vi "ParseMessage.vi"(11 "message in":string) -> (0 "Message type out":T1, 2 "Filename":string, 3 "message/data out":string)   [LabVIEW 2023, in "TCP_Server_Connection_Handler.lvlib" / "TCP_Server_Connection_Handler.lvclass"]
uses:
  TCP_Server_Connection_Handler.lvclass
  TCP_Server_Connection_Handler.lvclass/TCP_Server_Connection_Handler.ctl
  TypeDefinitions/messageType.ctl
  TCP_Server_Connection_Handler.lvlib
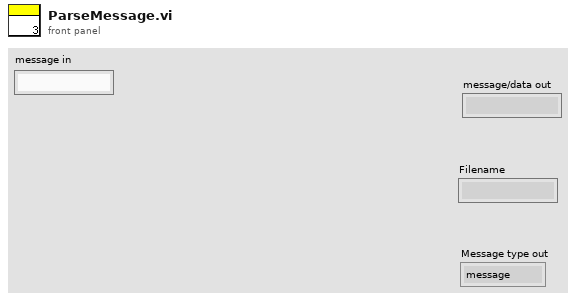
[diagram p1: front panel]
types:
  T1 = typedef "TCP_Server_Connection_Handler.lvlib/messageType.ctl" = enum16{"message", "file", "get", "ShutDown"}
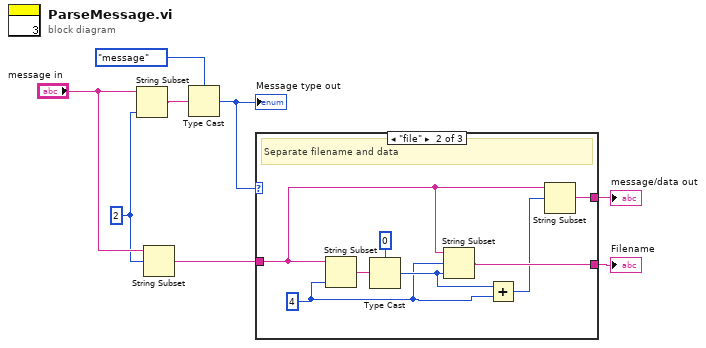
[diagram p0: block diagram]
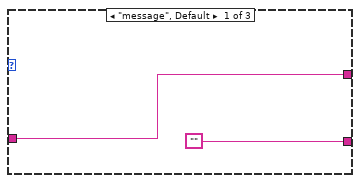
[diagram p2: hidden frame]
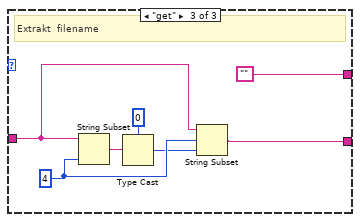
[diagram p3: hidden frame]
diagram:
  w2 = 2 ("length (rest)")
  n1 = String Subset(string="message in", length (rest)=w2) -> (substring=w5:string)  [unwired: 1 in]
  n2 = String Subset(string="message in", offset (0)=w2) -> (substring=w1:string)  [unwired: 1 in]
  n3 = Type Cast(type=messageType."message" ("MessageType"), x=w5) -> (*(type *) &x=w3:T1)
  "Message type out" <- w3
  n4 = case shown="\"file\"" w3 {
    tunnel: w1 -> [w9 w13 w21]
    tunnel: ["" w16 w23] -> w6
    tunnel: [w9 w11 ""] -> w7
    frame "message", Default {
    }
    frame "file" {
      w14 = 4 ("length (rest)")
      # "Separate filename and data"
      n5 = String Subset(string=w13, length (rest)=w14) -> (substring=w18:string)  [unwired: 1 in]
      n6 = Type Cast(type=0, x=w18) -> (*(type *) &x=w15:i32)
      n7 = String Subset(string=w13, offset (0)=w14, length (rest)=w15) -> (substring=w16:string)
      n8 = Add(x=w15, y=w14) -> (x+y=w12:i32)
      n9 = String Subset(string=w13, offset (0)=w12) -> (substring=w11:string)  [unwired: 1 in]
    }
    frame "get" {
      w22 = 4 ("length (rest)")
      # "Extrakt  filename"
      n10 = String Subset(string=w21, length (rest)=w22) -> (substring=w25:string)  [unwired: 1 in]
      n11 = Type Cast(type=0, x=w25) -> (*(type *) &x=w20:i32)
      n12 = String Subset(string=w21, offset (0)=w22, length (rest)=w20) -> (substring=w23:string)
    }
  }
  "message/data out" <- w7
  "Filename" <- w6
